vi "Store Configuration Parameters.vi"(8 "error in (no error)":errorcluster, 10 "refnum":T1, 11 "HW with output config in":refnum<class "HW with output config.lvclass">) -> (0 "error out":errorcluster, 2 "refnum out":T1, 3 "HW with output config out":refnum<class "HW with output config.lvclass">)   [LabVIEW 2017, in "Hardware.lvlib" / "HW with output config.lvclass"]
uses:
  HW with output config.lvclass
  C:/Program Files (x86)/National Instruments/LabVIEW 2017/user.lib/Configuration Dialog Actor/Configuration.lvclass
  <vilib>/Utility/config.llb/Config Data RefNum.ctl
  <userlib>/Configuration Dialog Actor/Configuration.lvclass/Configuration.ctl
  HW with output config.lvclass/HW with output config.ctl
  HW Config/HW Configuration.lvclass
  <userlib>/Configuration Dialog Actor/Configuration.lvclass
  <vilib>/Utility/config.llb/NI_LVConfig.lvlib
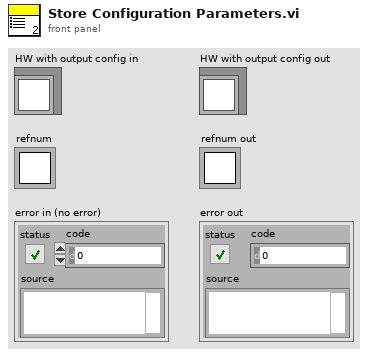
[diagram p1: front panel]
types:
  T1 = typedef "NI_LVConfig.lvlib/Config Data RefNum.ctl" = refnum<k1>
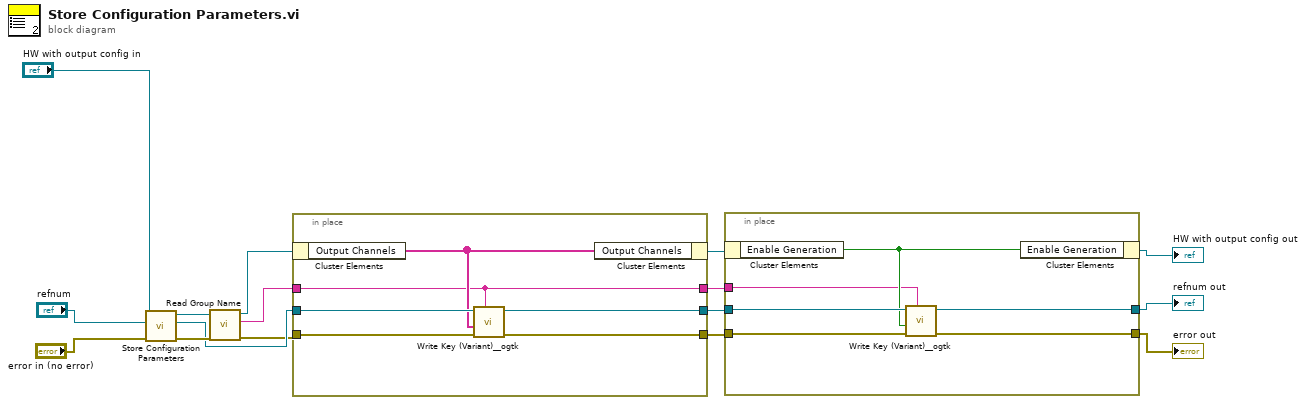
[diagram p0: block diagram]
diagram:
  n1 = call-parent "Store Configuration Parameters.vi"("error in (no error)"="error in (no error)", "refnum"="refnum", "HW Configuration in"="HW with output config in") -> ("error out"=w14:errorcluster, "refnum out"=w13:T1, "HW Configuration out"=w15:refnum<class "HW with output config.lvclass">)  [unwired: 6 in]
  n2 = call <userlib>:"Read Group Name.vi"("error in (no error)"=w14, "Configuration in"=w15) -> ("error out"=w12:errorcluster, "Group Name"=w11:string, "Configuration out"=w16:refnum<class "HW with output config.lvclass">)  [unwired: 7 in]
  n3 = in-place {
    in-place-border: w13 -> [w22]
    in-place-border: [w21] -> w5
    in-place-border: [w20] -> w4
    in-place-border: w12 -> [w18]
    in-place-border: w11 -> [w17]
    in-place-border: [w17] -> w10
    n4 = in-place-cluster #1(w16) -> ("Output Channels"=w19:string[])
    n5 = call <userlib>:"Write Key (Variant)__ogtk.vi"("section"=w17, "error in (no error)"=w18, "key-value"=w19, "refnum"=w22) -> ("error out"=w20:errorcluster, "refnum out"=w21:T1)  [unwired: 6 in]
    n6 = in-place-cluster #1("Output Channels"=w19) -> (w6:refnum<class "HW with output config.lvclass">)
  }
  n7 = in-place {
    in-place-border: w5 -> [w28]
    in-place-border: [w27] -> w2
    in-place-border: [w26] -> w1
    in-place-border: w4 -> [w24]
    in-place-border: w10 -> [w23]
    n8 = in-place-cluster #2(w6) -> ("Enable Generation"=w25:bool)
    n9 = call <userlib>:"Write Key (Variant)__ogtk.vi"("section"=w23, "error in (no error)"=w24, "key-value"=w25, "refnum"=w28) -> ("error out"=w26:errorcluster, "refnum out"=w27:T1)  [unwired: 6 in]
    n10 = in-place-cluster #2("Enable Generation"=w25) -> (→"HW with output config out":refnum<class "HW with output config.lvclass">)
  }
  "error out" <- w1
  "refnum out" <- w2
